vi "NMLWSD_Stability_Data_Collection.vi"() -> ()   [LabVIEW 2017]
uses:
  C:/Program Files (x86)/Newport/Newport USB Driver/Bin/UsbDllWrap.dll
  Program Files (x86)/Newport/Newport USB Driver/Bin/UsbDllWrap.dll
  <vilib>/Analysis/baseanly.llb/Mean (DBL).vi
  <vilib>/Utility/file.llb/Write Delimited Spreadsheet (string).vi
  <vilib>/Analysis/NI_AALBase.lvlib
panel:
  in  "Time":refnum<vi>
  in  "Date":refnum<vi>
  in  "Bytes Received":refnum<vi>
  in  "Module Error":refnum<vi>
  in  "Read Buffer":refnum<vi>
  out "read buffer":string
  in  "Error Log Msg":refnum<vi>
  out "System Data Array":dbl[][](array[numeric])
  out "MCU Data Array":dbl[][](array[numeric])
  in  "Data Error":refnum<vi>
  in  "TimeOut Error":refnum<vi>
  in  "Status Msg":refnum<vi>
  in  "Shutter Closed":refnum<vi>
  in  "Shutter Opened":refnum<vi>
  in  "Active UUT COMs":refnum<visa-resource-name>[](array[refnum])
  in  "Power Meter Ref":refnum<k24>
  out "Shtr Close":bool
  out "Shtr Open":bool
  out "All Results":dbl[][][](array[numeric]) format="%8_4g"
  in  "Serial Number":string[](array[string])=["1"]
  in  "Tpass Shtr Open":bool
  out "Shtr Ref Time":timestamp
  out "TimeS":string caption="Time"
  out "DateS":string caption="Date"
  out "Msg":string="\n\r" caption="Status"
  out "Bytes Rcvd":u32=1000
  out "Module Error":bool[](array[boolean])
  out "Data Error":bool
  out "Timeout":bool
  out "Points":i32[](array[numeric])
  out "UUT Count":i32(ring)=1 items=["1"=1, "2"=2, "3"=3, "4"=4, "5"=5, "6"=6, "7"=7, "8"=8]
  out "error":errorcluster
  out "Data Time":timestamp
  out "Collect":bool
  out "Save":bool
  out "Update Graph":bool
  in  "cDAQ2":string
  in  "Meas N":i32
  in  "WL: NML Only":i32(ring) items=["Red Only", "IR"]
  in  "FW inTest":u16(ring) items=["WSD Board", "NML Board"]
  in  "Sys Criteria":string[][](array[string])
  in  "FW Criteria":string[][](array[string])
  in  "FW ID":string[](array[string])
  in  "FW Prm":string[](array[string])
  out "SysCheck":string[][](array[string])
  out "MCUCheck":string[][](array[string])
  out "SysTrue":bool[][](array[boolean])
  out "MCUTrue":bool[][](array[boolean])
  in  "Shtr Ctrl Close, Seconds":dbl=6.0 max=60.0 format="%.3f"
  in  "cDAQ1":string
  out "Error Log Msg":string
  out "work buffer":string
  in  "Log File":path=path "C:/Test/WSNM Stability/Log.txt"
  out "System Data":dbl[](array[numeric]) format="%#_5p"
  out "MCU Data":dbl[](array[numeric]) format="%#_5p"
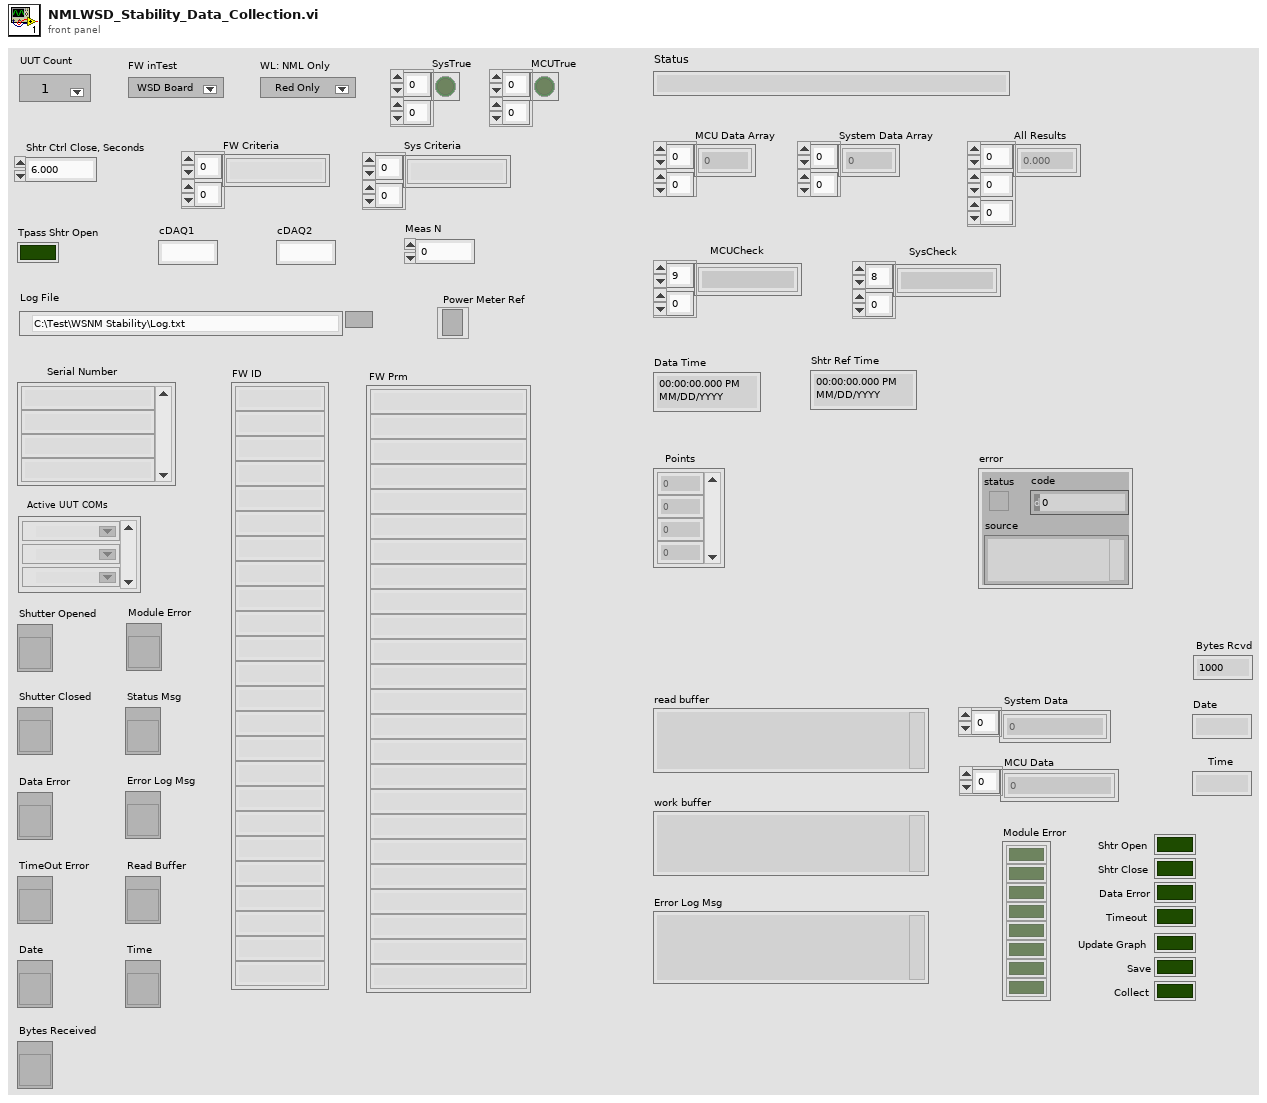
[diagram p1: front panel]
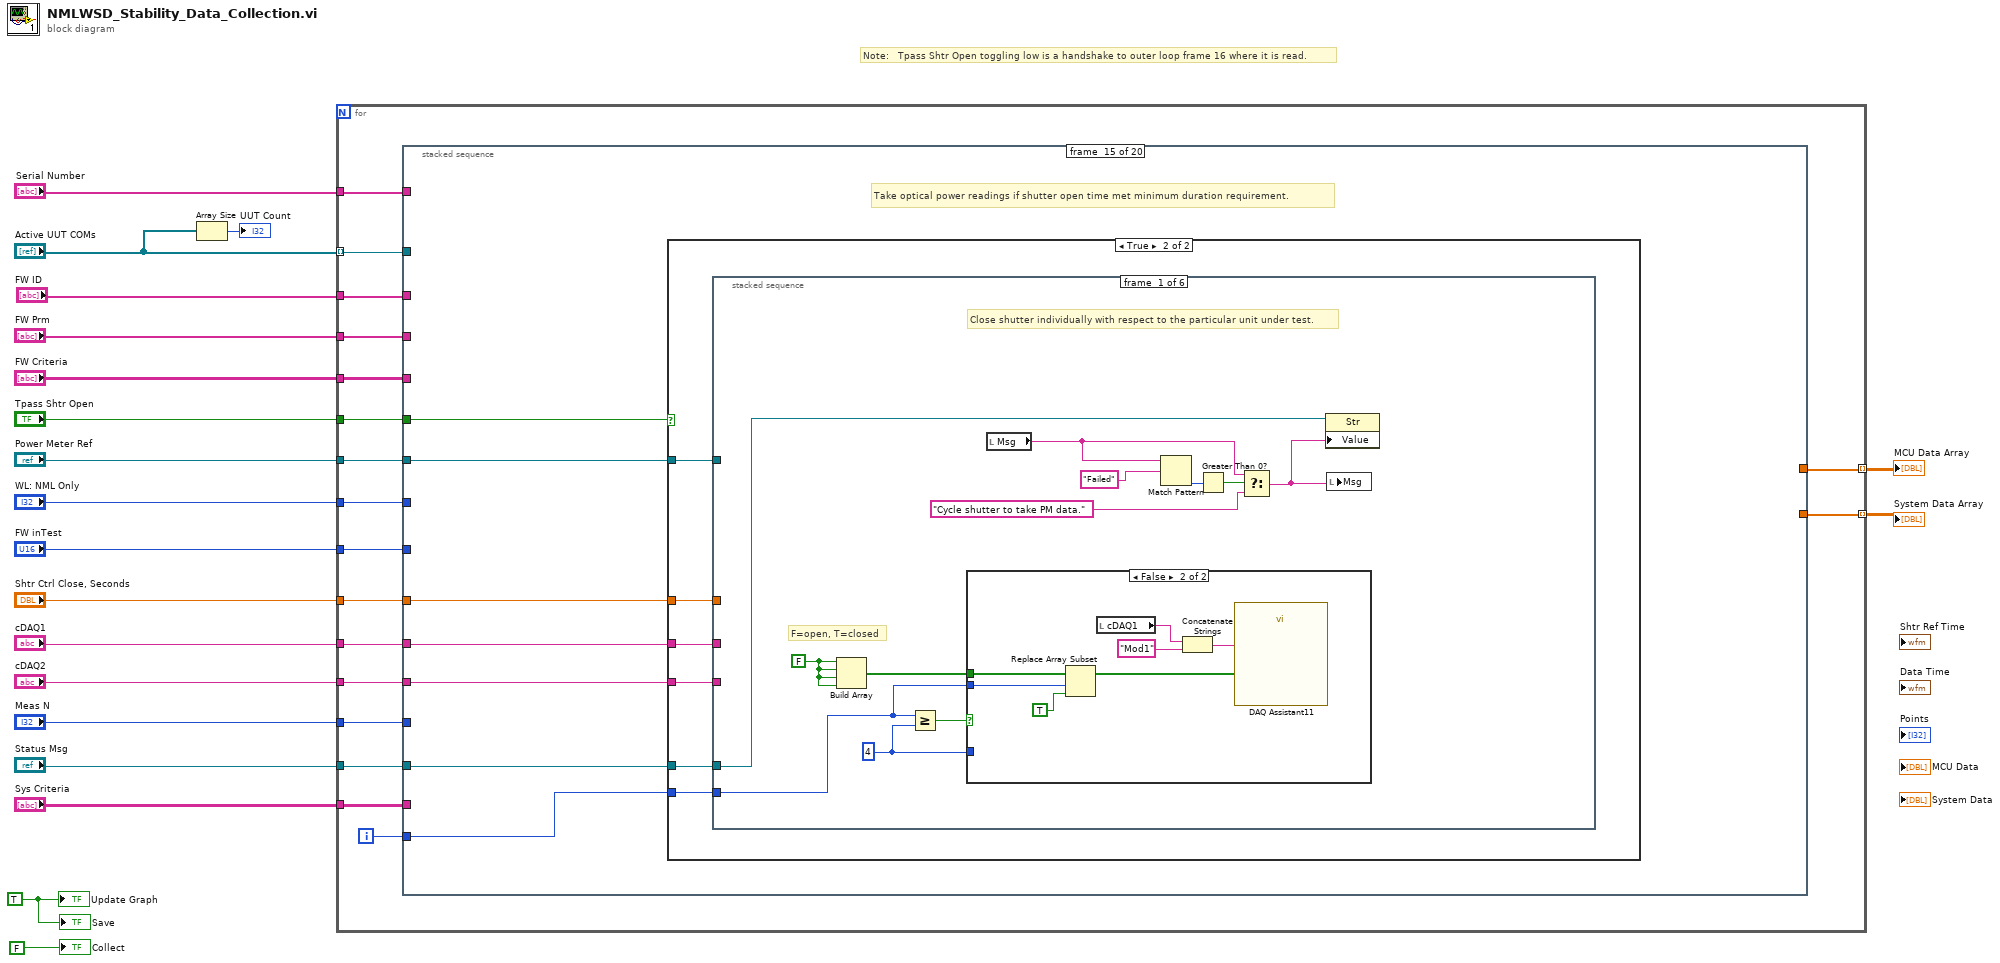
[diagram p0: block diagram]
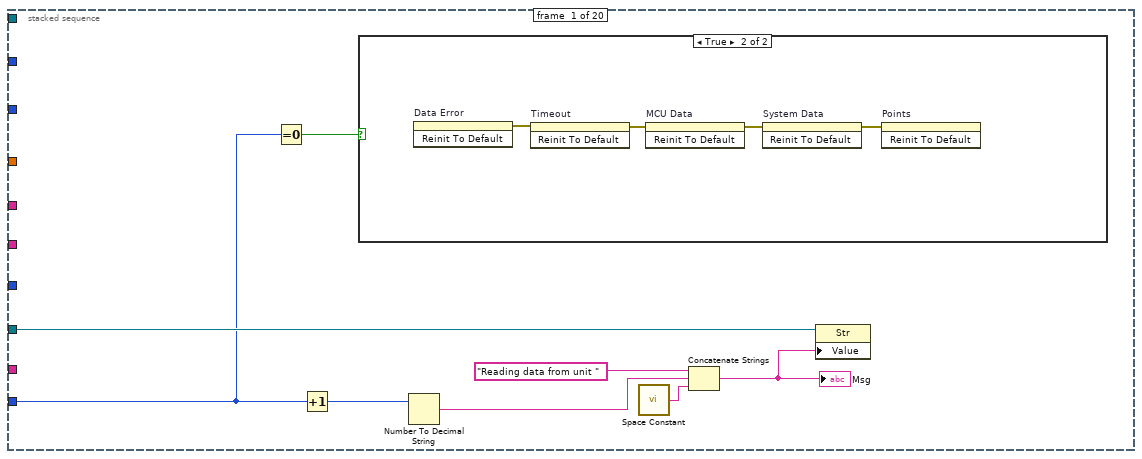
[diagram p2: hidden frame]
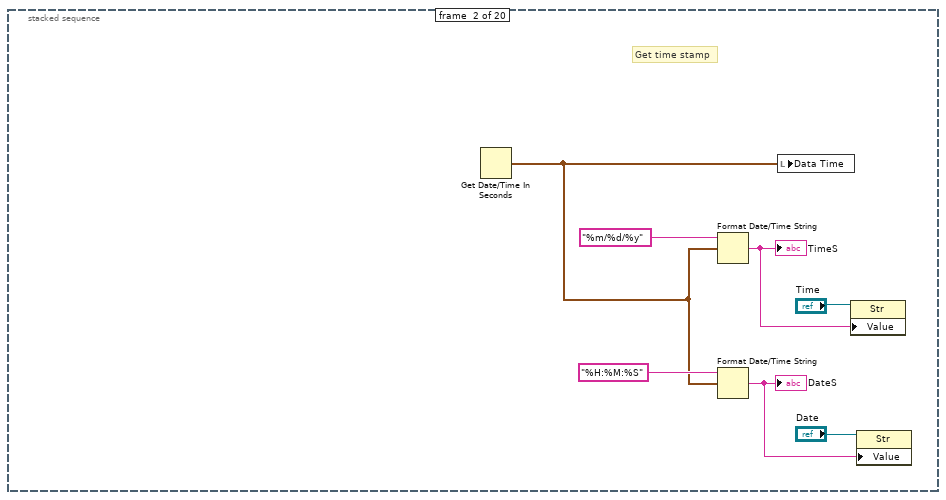
[diagram p4: hidden frame]
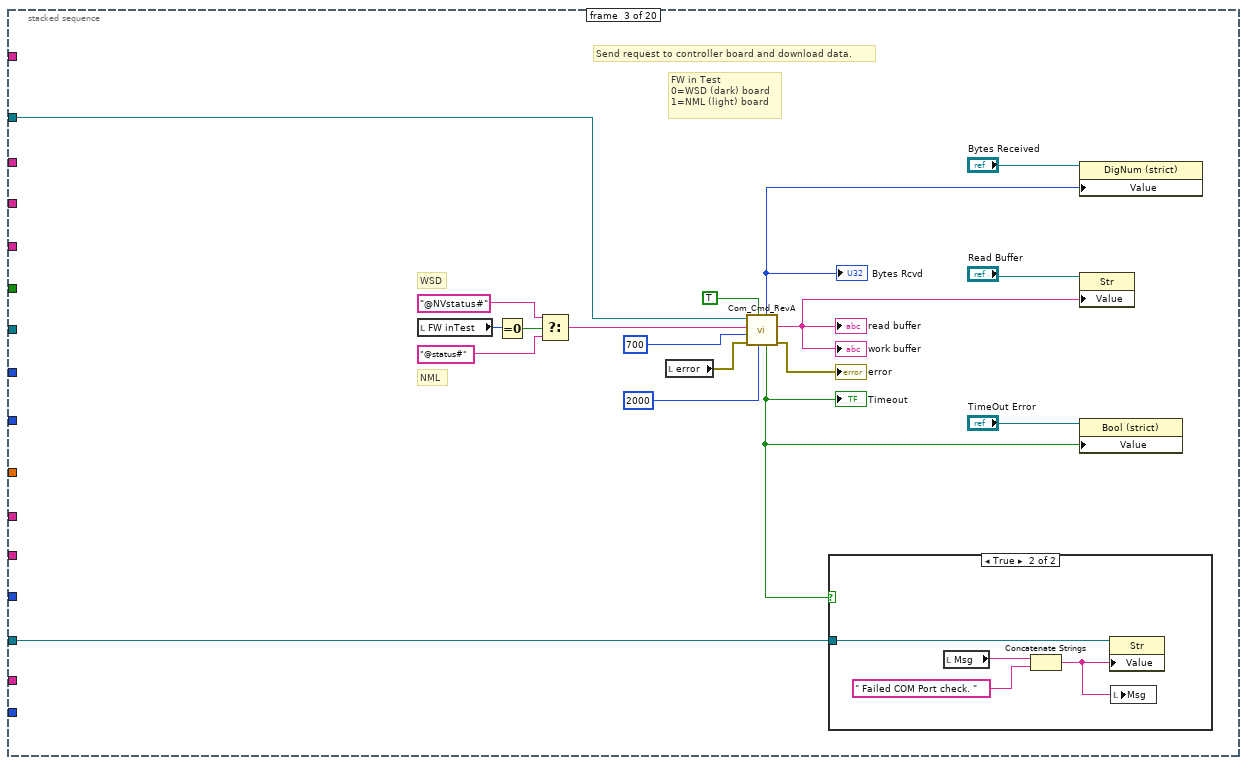
[diagram p5: hidden frame]
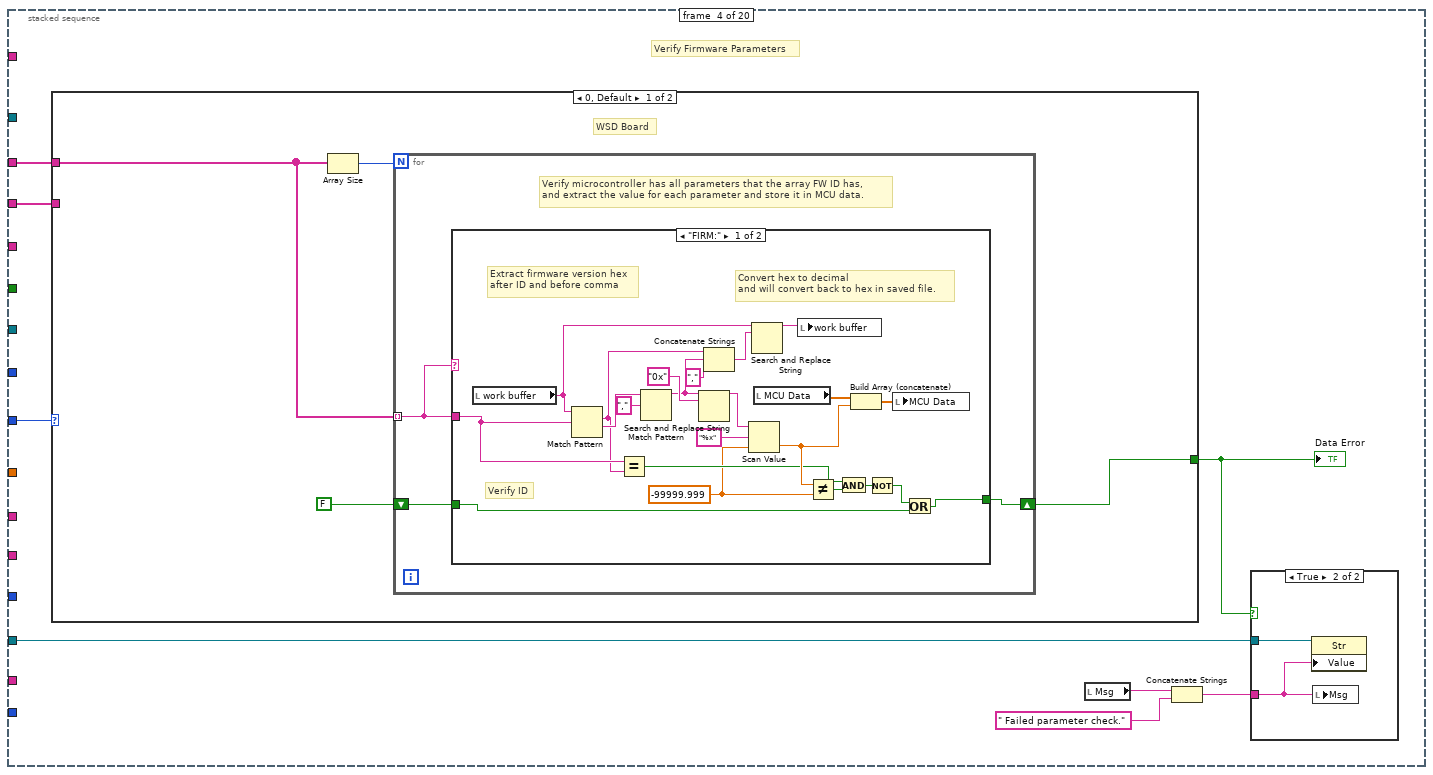
[diagram p7: hidden frame]
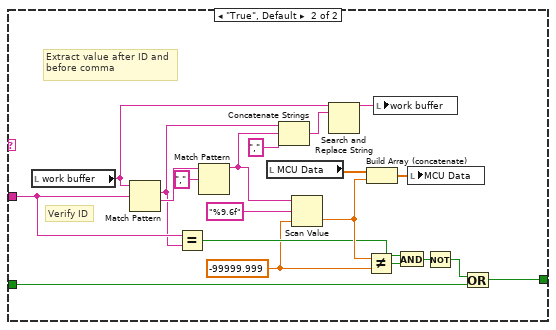
[diagram p9: hidden frame]
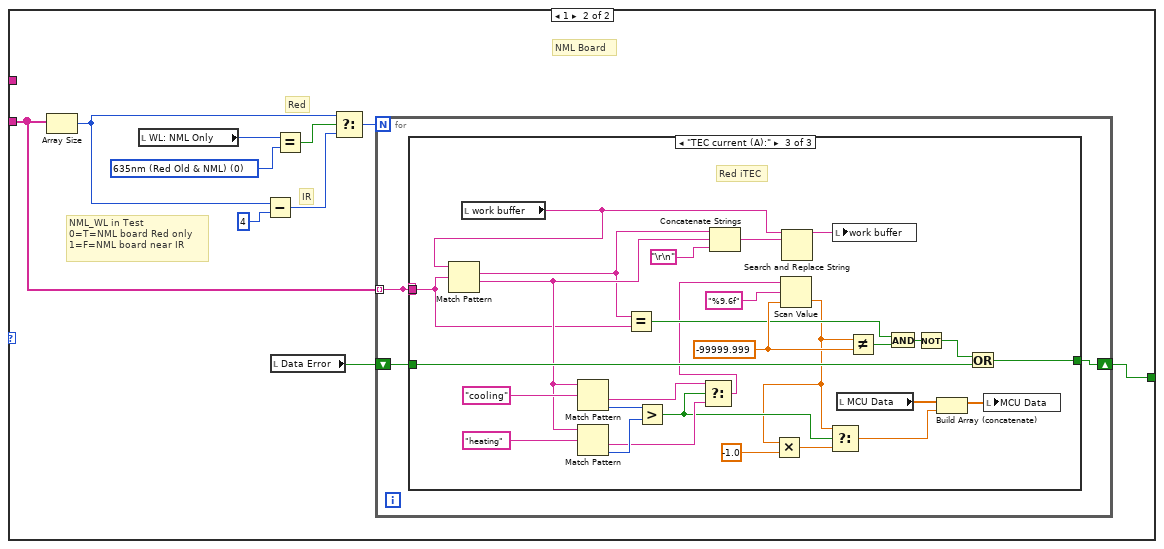
[diagram p10: hidden frame]
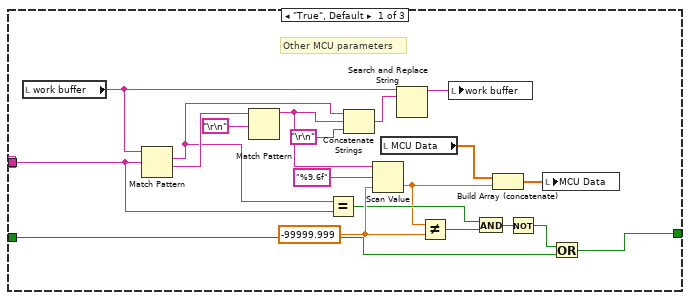
[diagram p11: hidden frame]
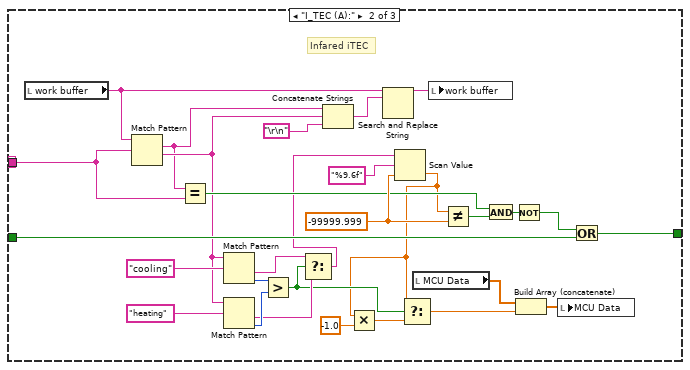
[diagram p12: hidden frame]
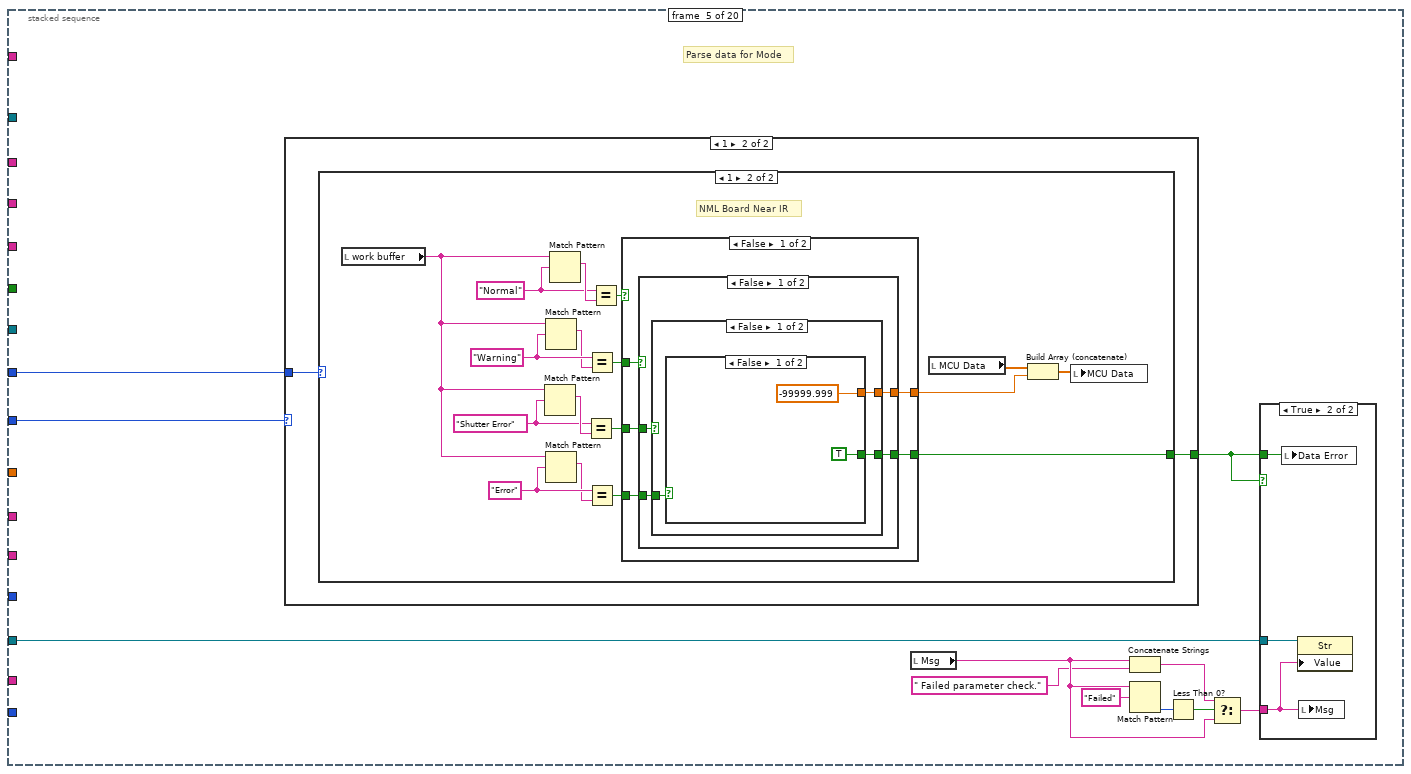
[diagram p13: hidden frame]
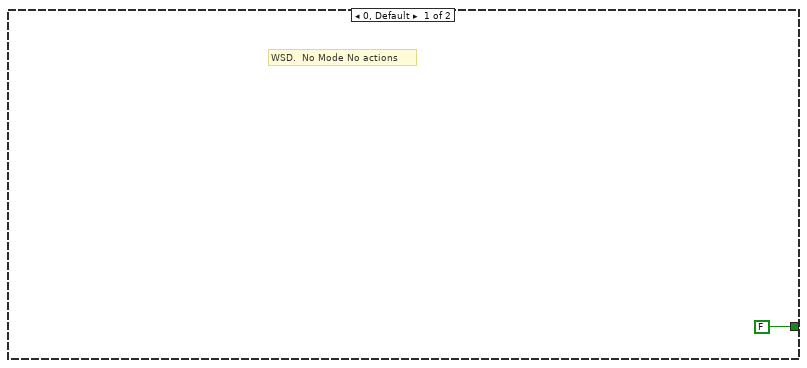
[diagram p15: hidden frame]
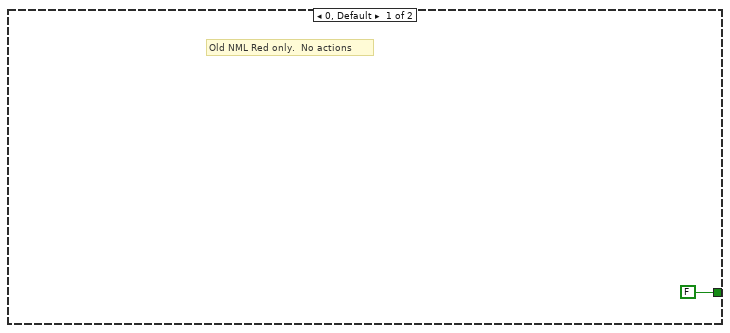
[diagram p16: hidden frame]
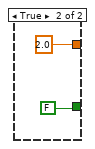
[diagram p17: hidden frame]
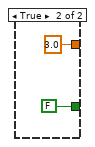
[diagram p18: hidden frame]
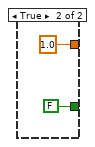
[diagram p19: hidden frame]
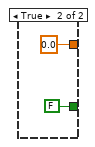
[diagram p20: hidden frame]
diagram:
  w20 = TRUE ("Update Graph")
  # "Note:   Tpass Shtr Open toggling low is a handshake to outer loop frame 16 where it is read."
  n1 = Array Size(array="Active UUT COMs") -> (size(s)=→"UUT Count":i32)
  n2 = for {
    tunnel: "Active UUT COMs" -> [w37] mode=indexing
    tunnel: "Power Meter Ref" -> [w36]
    tunnel: "Tpass Shtr Open" -> [w35]
    tunnel: "FW inTest" -> [w34]
    tunnel: "WL: NML Only" -> [w33]
    tunnel: "Shtr Ctrl Close, Seconds" -> [w32]
    tunnel: "cDAQ1" -> [w31]
    tunnel: "cDAQ2" -> [w30]
    tunnel: "FW ID" -> [w29]
    tunnel: "Meas N" -> [w28]
    tunnel: "Serial Number" -> [w27]
    tunnel: "Status Msg" -> [w26]
    tunnel: "Sys Criteria" -> [w25]
    tunnel: "FW Criteria" -> [w24]
    tunnel: [w23] -> w3 mode=indexing
    tunnel: [w22] -> w2 mode=indexing
    tunnel: "FW Prm" -> [w21]
    i -> [w38]
    n3 = stacked-sequence {
      tunnel: w38 -> [w43 _ _ _ _ _ _ w394 _ w442 _ _ _ w496 w573 w673 w693 w703 w744 _]
      tunnel: w37 -> [_ _ w65 _ _ _ _ _ _ _ _ _ _ _ _ _ _ _ _ _]
      tunnel: w36 -> [_ _ _ _ _ _ _ _ _ w441 _ _ _ _ w572 _ _ _ _ _]
      tunnel: w35 -> [_ _ _ _ _ _ _ _ _ _ _ _ _ _ w571 _ _ _ _ _]
      tunnel: w34 -> [_ _ _ w87 w240 w297 w354 _ _ _ _ _ _ _ _ _ _ _ _ _]
      tunnel: w33 -> [_ _ _ _ w239 w296 w353 _ _ _ _ _ _ _ _ _ _ _ _ _]
      tunnel: w32 -> [_ _ _ _ _ _ _ _ _ _ _ _ _ _ w570 _ _ _ _ _]
      tunnel: w31 -> [_ _ _ _ _ _ _ _ _ _ _ w471 _ _ w569 _ _ _ _ _]
      tunnel: w30 -> [_ _ _ _ _ _ _ _ _ _ _ _ _ _ w568 _ _ _ _ _]
      tunnel: w29 -> [_ _ _ w86 _ _ _ _ _ _ _ _ _ _ _ _ _ _ _ _]
      tunnel: w28 -> [_ _ _ _ _ _ _ _ _ _ _ _ _ _ _ w672 _ _ _ _]
      tunnel: w27 -> [_ _ _ _ _ _ _ w392 _ _ _ _ _ _ _ _ _ _ _ _]
      tunnel: w26 -> [w45 _ w63 w82 w232 w289 w346 _ w434 _ w465 _ w489 _ w567 _ _ _ _ _]
      tunnel: w25 -> [_ _ _ _ _ _ _ _ _ _ _ _ _ _ _ _ _ w702 _ _]
      tunnel: w24 -> [_ _ _ _ _ _ _ _ _ _ _ _ _ _ _ _ _ w701 _ _]
      tunnel: [_ _ _ _ _ _ _ _ _ _ _ _ _ _ _ _ w691 _ _ _] -> w23
      tunnel: [_ _ _ _ _ _ _ _ _ _ _ _ _ _ _ _ w690 _ _ _] -> w22
      tunnel: w21 -> [_ _ _ w80 _ _ _ _ _ _ _ _ _ _ _ _ _ _ _ _]
      frame #0 {
        n4 = Equal To 0?(x=w43) -> (x = 0?=w46:bool)
        n5 = Increment(x=w43) -> (x+1=w44:i32)
        n6 = case shown="True" w46 {
          frame False {
          }
          frame True {
            n7 = invoke on="Data Error" class="Bool (strict)" method="Reinit To Default"() -> (error out=w49:errorcluster)  [unwired: 3 in, 2 out]
            n8 = invoke on="Timeout" class="Bool (strict)" method="Reinit To Default"(error in=w49) -> (error out=w48:errorcluster)  [unwired: 2 in, 2 out]
            n9 = invoke on="MCU Data" class="Arr (strict)" method="Reinit To Default"(error in=w48) -> (error out=w50:errorcluster)  [unwired: 2 in, 2 out]
            n10 = invoke on="System Data" class="Arr (strict)" method="Reinit To Default"(error in=w50) -> (error out=w47:errorcluster)  [unwired: 2 in, 2 out]
            n11 = invoke on="Points" class="Arr (strict)" method="Reinit To Default"(error in=w47) -> ()  [unwired: 2 in, 3 out]
          }
        }
        n12 = Number To Decimal String(number=w44) -> (decimal integer string=w41:string)  [unwired: 1 in]
        n13 = call <vilib>:"Space Constant.vi"() -> ("String"=w39:string)
        n14 = Concatenate Strings("Reading data from unit " ("Msg"), w41, w39) -> (w40:string)
        "Msg" <- w40
        n15 = property class="Str"(reference=w45, "Value"=w40) -> ()  [unwired: 1 in, 2 out]
      }
      frame #1 {
        # "Get time stamp"
        n16 = Get Date/Time In Seconds() -> (seconds since 1Jan1904=w55:timestamp)
        n17 = Format Date/Time String(time format string (%c)="%m/%d/%y", seconds (now)=w55) -> (date/time string=w52:string)  [unwired: 1 in]
        "TimeS" <- w52
        n18 = Format Date/Time String(time format string (%c)="%H:%M:%S", seconds (now)=w55) -> (date/time string=w51:string)  [unwired: 1 in]
        "DateS" <- w51
        n19 = local write "Data Time"(w55) -> ()
        n20 = property class="Str"(reference="Time", "Value"=w52) -> ()  [unwired: 1 in, 2 out]
        n21 = property class="Str"(reference="Date", "Value"=w51) -> ()  [unwired: 1 in, 2 out]
      }
      frame #2 {
        # "NML"
        # "WSD"
        # "FW in Test\n0=WSD (dark) board\n1=NML (light) board"
        # "Send request to controller board and download data."
        n22 = local read "FW inTest"() -> (w68:u16)
        n23 = Equal To 0?(x=w68) -> (x = 0?=w67:bool)
        n24 = Select(t="@NVstatus#" ("string"), s=w67, f="@status#" ("string")) -> (s? t:f=w71:string)
        n25 = local read "error"() -> (w75:errorcluster)
        n26 = call "Com_Cmd_RevA.vi"("Timeout"=2000, "Query"=TRUE, "error in"=w75, "Delay, ms"=u32 700, "write buffer"=w71, "VISA"=w65) -> ("error out"=→"error":errorcluster, "read buffer"=w60:string, "Timeout"=w62:bool, "return count"=w58:u32)  [unwired: 2 out]
        "work buffer" <- w60
        "Timeout" <- w62
        "Bytes Rcvd" <- w58
        "read buffer" <- w60
        n27 = case shown="True" w62 {
          tunnel: w63 -> [_ w77]
          frame False {
          }
          frame True {
            n28 = local read "Msg"() -> (w79:string)
            n29 = Concatenate Strings(w79, " Failed COM Port check. " ("string")) -> (w76:string)
            n30 = property class="Str"(reference=w77, "Value"=w76) -> ()  [unwired: 1 in, 2 out]
            n31 = local write "Msg"(w76) -> ()
          }
        }
        n32 = property class="DigNum (strict)"(reference="Bytes Received", "Value"=w58) -> ()  [unwired: 1 in, 2 out]
        n33 = property class="Str"(reference="Read Buffer", "Value"=w60) -> ()  [unwired: 1 in, 2 out]
        n34 = property class="Bool (strict)"(reference="TimeOut Error", "Value"=w62) -> ()  [unwired: 1 in, 2 out]
      }
      frame #3 {
        # "Verify Firmware Parameters"
        n35 = case shown="0, Default" w87 {
          tunnel: w86 -> [w91 _]
          tunnel: [w90 w140] -> w85
          tunnel: w80 -> [_ w139]
          frame 0, Default {
            # "WSD Board"
            n36 = Array Size(array=w91) -> (size(s)=w92:i32)
            n37 = for {
              N: w92 -> [_]
              shift-right: [w95] -> w90
              shift-left: FALSE ("Data Err") -> [w96]
              tunnel: w91 -> [w94] mode=indexing
              # "Verify microcontroller has all parameters that the array FW ID has,\nand extract the value for each parameter and store it in MCU data."
              n38 = case shown="\"FIRM:\"" w94 {
                tunnel: w94 -> [w105 w125]
                tunnel: w96 -> [w107 w138]
                tunnel: [w106 w137] -> w95
                frame "FIRM:" {
                  w111 = -99999.999 ("default (0 dbl)")
                  # "Convert hex to decimal\nand will convert back to hex in saved file."
                  # "Extract firmware version hex\nafter ID and before comma"
                  # "Verify ID"
                  n39 = local read "work buffer"() -> (w99:string)
                  n40 = Match Pattern(string=w99, regular expression=w105) -> (match substring=w102:string, after substring=w109:string)  [unwired: 1 in, 2 out]
                  n41 = Equal?(x=w105, y=w102) -> (x = y?=w113:bool)
                  n42 = Match Pattern(string=w109, regular expression=",") -> (before substring=w101:string)  [unwired: 1 in, 3 out]
                  n43 = Search and Replace String(input string=w101, search string="0x") -> (result string=w103:string)  [unwired: 6 in, 3 out]
                  n44 = Concatenate Strings(w102, w101, "," ("string")) -> (w98:string)
                  n45 = Scan Value(string=w103, format string="%x", default (0 dbl)=w111) -> (value=w116:dbl)  [unwired: 1 out]
                  n46 = Search and Replace String(input string=w99, search string=w98) -> (result string=w97:string)  [unwired: 6 in, 3 out]
                  n47 = local read "MCU Data"() -> (w114:dbl[])
                  n48 = local write "work buffer"(w97) -> ()
                  n49 = Not Equal?(x=w116, y=w111) -> (x != y?=w112:bool)
                  n50 = And(x=w113, y=w112) -> (x .and. y?=w117:bool)
                  n51 = Build Array (concatenate)(w114, w116) -> (w115:dbl[])
                  n52 = Not(x=w117) -> (.not. x?=w118:bool)
                  n53 = local write "MCU Data"(w115) -> ()
                  n54 = Or(x=w118, y=w107) -> (x .or. y?=w106:bool)
                }
                frame "True", Default {
                  w129 = -99999.999 ("default (0 dbl)")
                  # "Extract value after ID and\nbefore comma"
                  # "Verify ID"
                  n55 = local read "work buffer"() -> (w121:string)
                  n56 = Match Pattern(string=w121, regular expression=w125) -> (match substring=w123:string, after substring=w127:string)  [unwired: 1 in, 2 out]
                  n57 = Equal?(x=w125, y=w123) -> (x = y?=w131:bool)
                  n58 = Match Pattern(string=w127, regular expression=",") -> (before substring=w122:string)  [unwired: 1 in, 3 out]
                  n59 = local read "MCU Data"() -> (w132:dbl[])
                  n60 = Concatenate Strings(w123, w122, "," ("string")) -> (w120:string)
                  n61 = Scan Value(string=w122, format string="%9.6f", default (0 dbl)=w129) -> (value=w134:dbl)  [unwired: 1 out]
                  n62 = Search and Replace String(input string=w121, search string=w120) -> (result string=w119:string)  [unwired: 6 in, 3 out]
                  n63 = Not Equal?(x=w134, y=w129) -> (x != y?=w130:bool)
                  n64 = Build Array (concatenate)(w132, w134) -> (w133:dbl[])
                  n65 = local write "work buffer"(w119) -> ()
                  n66 = And(x=w131, y=w130) -> (x .and. y?=w135:bool)
                  n67 = local write "MCU Data"(w133) -> ()
                  n68 = Not(x=w135) -> (.not. x?=w136:bool)
                  n69 = Or(x=w136, y=w138) -> (x .or. y?=w137:bool)
                }
              }
            }
          }
          frame 1 {
            w142 = 0 items=["635nm (Red Old & NML)", "Red-780-850nm (IR NewNML FW)", "Mix NML FW"] ("Color")
            # "NML Board"
            # "NML_WL in Test\n0=T=NML board Red only\n1=F=NML board near IR"
            # "IR"
            # "Red"
            n70 = Array Size(array=w139) -> (size(s)=w146:i32)
            n71 = local read "WL: NML Only"() -> (w143:i32)
            n72 = Subtract(x=w146, y=4) -> (x-y=w144:i32)
            n73 = local read "Data Error"() -> (w141:bool)
            n74 = Equal?(x=w143, y=w142) -> (x = y?=w148:bool)
            n75 = Select(t=w146, s=w148, f=w144) -> (s? t:f=w147:i32)
            n76 = for {
              N: w147 -> [_]
              tunnel: w139 -> [w149] mode=indexing
              shift-right: [w150] -> w140
              shift-left: w141 -> [w151]
              n77 = case shown="\"TEC current (A):\"" w149 {
                tunnel: w151 -> [w162 w192 w221]
                tunnel: [w161 w191 w220] -> w150
                tunnel: w149 -> [w153 w172 w202]
                frame "True", Default {
                  w170 = -99999.999 ("default (0 dbl)")
                  # "Other MCU parameters"
                  n78 = local read "work buffer"() -> (w152:string)
                  n79 = Match Pattern(string=w152, regular expression=w153) -> (match substring=w154:string, after substring=w159:string)  [unwired: 1 in, 2 out]
                  n80 = Match Pattern(string=w159, regular expression="\r\n") -> (before substring=w157:string)  [unwired: 1 in, 3 out]
                  n81 = Equal?(x=w154, y=w153) -> (x = y?=w168:bool)
                  n82 = Concatenate Strings(w154, w157, "\r\n") -> (w156:string)
                  n83 = Scan Value(string=w157, format string="%9.6f", default (0 dbl)=w170) -> (value=w165:dbl)  [unwired: 1 out]
                  n84 = local read "MCU Data"() -> (w167:dbl[])
                  n85 = Search and Replace String(input string=w152, search string=w156) -> (result string=w155:string)  [unwired: 6 in, 3 out]
                  n86 = Not Equal?(x=w165, y=w170) -> (x != y?=w169:bool)
                  n87 = local write "work buffer"(w155) -> ()
                  n88 = And(x=w168, y=w169) -> (x .and. y?=w164:bool)
                  n89 = Build Array (concatenate)(w167, w165) -> (w166:dbl[])
                  n90 = Not(x=w164) -> (.not. x?=w163:bool)
                  n91 = local write "MCU Data"(w166) -> ()
                  n92 = Or(x=w163, y=w162) -> (x .or. y?=w161:bool)
                }
                frame "I_TEC (A):" {
                  w199 = -99999.999 ("default (0 dbl)")
                  # "Infared iTEC"
                  n93 = local read "work buffer"() -> (w176:string)
                  n94 = Match Pattern(string=w176, regular expression=w172) -> (match substring=w173:string, after substring=w174:string)  [unwired: 1 in, 2 out]
                  n95 = Equal?(x=w173, y=w172) -> (x = y?=w197:bool)
                  n96 = Match Pattern(string=w174, regular expression="cooling") -> (after substring=w186:string, offset past match=w188:i32)  [unwired: 1 in, 2 out]
                  n97 = Match Pattern(string=w174, regular expression="heating") -> (after substring=w185:string, offset past match=w187:i32)  [unwired: 1 in, 2 out]
                  n98 = Greater?(x=w188, y=w187) -> (0:w184:bool)
                  n99 = Select(t=w186, s=w184, f=w185) -> (s? t:f=w175:string)
                  n100 = Concatenate Strings(w173, w174, "\r\n") -> (w179:string)
                  n101 = Search and Replace String(input string=w176, search string=w179) -> (result string=w178:string)  [unwired: 6 in, 3 out]
                  n102 = Scan Value(string=w175, format string="%9.6f", default (0 dbl)=w199) -> (value=w181:dbl)  [unwired: 1 out]
                  n103 = Multiply(x=w181, y=-1.0) -> (x*y=w182:dbl)
                  n104 = Select(t=w181, s=w184, f=w182) -> (s? t:f=w180:dbl)
                  n105 = local read "MCU Data"() -> (w196:dbl[])
                  n106 = local write "work buffer"(w178) -> ()
                  n107 = Not Equal?(x=w181, y=w199) -> (x != y?=w198:bool)
                  n108 = And(x=w197, y=w198) -> (x .and. y?=w194:bool)
                  n109 = Not(x=w194) -> (.not. x?=w193:bool)
                  n110 = Build Array (concatenate)(w196, w180) -> (w195:dbl[])
                  n111 = local write "MCU Data"(w195) -> ()
                  n112 = Or(x=w193, y=w192) -> (x .or. y?=w191:bool)
                }
                frame "TEC current (A):" {
                  w228 = -99999.999 ("default (0 dbl)")
                  # "Red iTEC"
                  n113 = local read "work buffer"() -> (w204:string)
                  n114 = Match Pattern(string=w204, regular expression=w202) -> (match substring=w201:string, after substring=w203:string)  [unwired: 1 in, 2 out]
                  n115 = Match Pattern(string=w203, regular expression="cooling") -> (after substring=w215:string, offset past match=w217:i32)  [unwired: 1 in, 2 out]
                  n116 = Match Pattern(string=w203, regular expression="heating") -> (after substring=w214:string, offset past match=w216:i32)  [unwired: 1 in, 2 out]
                  n117 = Equal?(x=w201, y=w202) -> (x = y?=w226:bool)
                  n118 = Greater?(x=w217, y=w216) -> (0:w212:bool)
                  n119 = Select(t=w215, s=w212, f=w214) -> (s? t:f=w213:string)
                  n120 = Concatenate Strings(w201, w203, "\r\n") -> (w207:string)
                  n121 = Scan Value(string=w213, format string="%9.6f", default (0 dbl)=w228) -> (value=w209:dbl)  [unwired: 1 out]
                  n122 = Multiply(x=w209, y=-1.0) -> (x*y=w210:dbl)
                  n123 = Search and Replace String(input string=w204, search string=w207) -> (result string=w206:string)  [unwired: 6 in, 3 out]
                  n124 = Select(t=w209, s=w212, f=w210) -> (s? t:f=w208:dbl)
                  n125 = local write "work buffer"(w206) -> ()
                  n126 = local read "MCU Data"() -> (w225:dbl[])
                  n127 = Not Equal?(x=w209, y=w228) -> (x != y?=w227:bool)
                  n128 = And(x=w226, y=w227) -> (x .and. y?=w223:bool)
                  n129 = Not(x=w223) -> (.not. x?=w222:bool)
                  n130 = Build Array (concatenate)(w225, w208) -> (w224:dbl[])
                  n131 = Or(x=w222, y=w221) -> (x .or. y?=w220:bool)
                  n132 = local write "MCU Data"(w224) -> ()
                }
              }
            }
          }
        }
        "Data Error" <- w85
        n133 = local read "Msg"() -> (w84:string)
        n134 = Concatenate Strings(w84, " Failed parameter check." ("string")) -> (w81:string)
        n135 = case shown="True" w85 {
          tunnel: w82 -> [_ w89]
          tunnel: w81 -> [_ w88]
          frame False {
          }
          frame True {
            n136 = property class="Str"(reference=w89, "Value"=w88) -> ()  [unwired: 1 in, 2 out]
            n137 = local write "Msg"(w88) -> ()
          }
        }
      }
      frame #4 {
        # "Parse data for Mode"
        n138 = case shown="1" w240 {
          tunnel: w239 -> [_ w246]
          tunnel: [FALSE w245] -> w231
          frame 0, Default {
            # "WSD.  No Mode No actions"
          }
          frame 1 {
            n139 = case shown="1" w246 {
              tunnel: [FALSE w248] -> w245
              frame 0, Default {
                # "Old NML Red only.  No actions"
              }
              frame 1 {
                w256 = "Error" ("regular expression")
                w257 = "Shutter Error" ("regular expression")
                w260 = "Warning" ("regular expression")
                w261 = "Normal" ("regular expression")
                # "NML Board Near IR"
                n140 = local read "work buffer"() -> (w254:string)
                n141 = Match Pattern(string=w254, regular expression=w257) -> (match substring=w258:string)  [unwired: 1 in, 3 out]
                n142 = Match Pattern(string=w254, regular expression=w260) -> (match substring=w259:string)  [unwired: 1 in, 3 out]
                n143 = Match Pattern(string=w254, regular expression=w256) -> (match substring=w255:string)  [unwired: 1 in, 3 out]
                n144 = Match Pattern(string=w254, regular expression=w261) -> (match substring=w264:string)  [unwired: 1 in, 3 out]
                n145 = Equal?(x=w257, y=w258) -> (x = y?=w250:bool)
                n146 = Equal?(x=w260, y=w259) -> (x = y?=w251:bool)
                n147 = Equal?(x=w256, y=w255) -> (x = y?=w249:bool)
                n148 = Equal?(x=w261, y=w264) -> (x = y?=w253:bool)
                n149 = case shown="False" w253 {
                  tunnel: [w268 0.0] -> w252
                  tunnel: w251 -> [w269 _]
                  tunnel: w250 -> [w267 _]
                  tunnel: w249 -> [w266 _]
                  tunnel: [w265 FALSE] -> w248
                  frame False {
                    n150 = case shown="False" w269 {
                      tunnel: [w272 1.0] -> w268
                      tunnel: w267 -> [w273 _]
                      tunnel: w266 -> [w271 _]
                      tunnel: [w270 FALSE] -> w265
                      frame False {
                        n151 = case shown="False" w273 {
                          tunnel: [w275 3.0] -> w272
                          tunnel: w271 -> [w276 _]
                          tunnel: [w274 FALSE] -> w270
                          frame False {
                            n152 = case shown="False" w276 {
                              tunnel: [-99999.999 ("default (0 dbl)") 2.0] -> w275
                              tunnel: [TRUE ("Data Err") FALSE] -> w274
                              frame False {
                              }
                              frame True {
                              }
                            }
                          }
                          frame True {
                          }
                        }
                      }
                      frame True {
                      }
                    }
                  }
                  frame True {
                  }
                }
                n153 = local read "MCU Data"() -> (w263:dbl[])
                n154 = Build Array (concatenate)(w263, w252) -> (w262:dbl[])
                n155 = local write "MCU Data"(w262) -> ()
              }
            }
          }
        }
        n156 = local read "Msg"() -> (w237:string)
        n157 = Concatenate Strings(w237, " Failed parameter check." ("string")) -> (w236:string)
        n158 = Match Pattern(string=w237, regular expression="Failed") -> (offset past match=w234:i32)  [unwired: 1 in, 3 out]
        n159 = Less Than 0?(x=w234) -> (x < 0?=w235:bool)
        n160 = Select(t=w236, s=w235, f=w237) -> (s? t:f=w238:string)
        n161 = case shown="True" w231 {
          tunnel: w232 -> [_ w243]
          tunnel: w238 -> [_ w242]
          tunnel: w231 -> [_ w241]
          frame False {
          }
          frame True {
            n162 = local write "Data Error"(w241) -> ()
            n163 = property class="Str"(reference=w243, "Value"=w242) -> ()  [unwired: 1 in, 2 out]
            n164 = local write "Msg"(w242) -> ()
          }
        }
      }
      frame #5 {
        # "Parse data for wavelength."
        n165 = case shown="1" w297 {
          tunnel: w296 -> [_ w303]
          tunnel: [FALSE w302] -> w288
          frame 0, Default {
            # "WSD.  No Mode No actions"
          }
          frame 1 {
            # "NML_WL in Test\n0=T=NML board Red only\n1=F=NML board near IR"
            # "NML"
            n166 = case shown="1" w303 {
              tunnel: [FALSE w305] -> w302
              frame 0, Default {
                # "Old NML Red only.  No actions"
              }
              frame 1 {
                w313 = "850" ("regular expression")
                w314 = "780" ("regular expression")
                w317 = "Red" ("regular expression")
                w318 = "None" ("regular expression")
                # "NML IR"
                n167 = local read "work buffer"() -> (w311:string)
                n168 = Match Pattern(string=w311, regular expression=w314) -> (match substring=w315:string)  [unwired: 1 in, 3 out]
                n169 = Match Pattern(string=w311, regular expression=w317) -> (match substring=w316:string)  [unwired: 1 in, 3 out]
                n170 = Match Pattern(string=w311, regular expression=w313) -> (match substring=w312:string)  [unwired: 1 in, 3 out]
                n171 = Match Pattern(string=w311, regular expression=w318) -> (match substring=w321:string)  [unwired: 1 in, 3 out]
                n172 = Equal?(x=w314, y=w315) -> (x = y?=w307:bool)
                n173 = Equal?(x=w317, y=w316) -> (x = y?=w308:bool)
                n174 = Equal?(x=w313, y=w312) -> (x = y?=w306:bool)
                n175 = Equal?(x=w318, y=w321) -> (x = y?=w310:bool)
                n176 = case shown="False" w310 {
                  tunnel: [w325 0.0] -> w309
                  tunnel: w308 -> [w326 _]
                  tunnel: w307 -> [w324 _]
                  tunnel: w306 -> [w323 _]
                  tunnel: [w322 FALSE] -> w305
                  frame False {
                    n177 = case shown="False" w326 {
                      tunnel: [w329 1.0] -> w325
                      tunnel: w324 -> [w330 _]
                      tunnel: w323 -> [w328 _]
                      tunnel: [w327 FALSE] -> w322
                      frame False {
                        n178 = case shown="False" w330 {
                          tunnel: [w332 2.0] -> w329
                          tunnel: w328 -> [w333 _]
                          tunnel: [w331 FALSE] -> w327
                          frame False {
                            n179 = case shown="False" w333 {
                              tunnel: [-99999.999 ("default (0 dbl)") 3.0] -> w332
                              tunnel: [TRUE ("Data Err") FALSE] -> w331
                              frame False {
                              }
                              frame True {
                              }
                            }
                          }
                          frame True {
                          }
                        }
                      }
                      frame True {
                      }
                    }
                  }
                  frame True {
                  }
                }
                n180 = local read "MCU Data"() -> (w320:dbl[])
                n181 = Build Array (concatenate)(w320, w309) -> (w319:dbl[])
                n182 = local write "MCU Data"(w319) -> ()
              }
            }
          }
        }
        n183 = local read "Msg"() -> (w291:string)
        n184 = Concatenate Strings(w291, " Failed parameter check." ("string")) -> (w292:string)
        n185 = Match Pattern(string=w291, regular expression="Failed") -> (offset past match=w295:i32)  [unwired: 1 in, 3 out]
        n186 = Less Than 0?(x=w295) -> (x < 0?=w293:bool)
        n187 = Select(t=w292, s=w293, f=w291) -> (s? t:f=w290:string)
        n188 = case shown="True" w288 {
          tunnel: w289 -> [_ w300]
          tunnel: w290 -> [_ w299]
          tunnel: w288 -> [_ w298]
          frame False {
          }
          frame True {
            n189 = local write "Data Error"(w298) -> ()
            n190 = property class="Str"(reference=w300, "Value"=w299) -> ()  [unwired: 1 in, 2 out]
            n191 = local write "Msg"(w299) -> ()
          }
        }
      }
      frame #6 {
        # "Parse Data for LHM Calibration Gain and Offset"
        n192 = case shown="1" w354 {
          tunnel: w353 -> [_ w360]
          tunnel: [FALSE w359] -> w345
          frame 0, Default {
            # "WSD.  No Mode No actions"
          }
          frame 1 {
            # "NML"
            n193 = case shown="1" w360 {
              tunnel: [FALSE w362] -> w359
              frame 0, Default {
                # "Old NML Red only.  No actions"
              }
              frame 1 {
                w363 = "LHM Calibration:" ("regular expression")
                w370 = -99999.999 ("default (0 dbl)")
                # "NML IR"
                n194 = local read "work buffer"() -> (w377:string)
                n195 = Match Pattern(string=w377, regular expression=w363) -> (match substring=w364:string, after substring=w378:string)  [unwired: 1 in, 2 out]
                n196 = Equal?(x=w364, y=w363) -> (x = y?=w383:bool)
                n197 = Match Pattern(string=w378, regular expression="Gain=") -> (after substring=w373:string)  [unwired: 1 in, 3 out]
                n198 = Match Pattern(string=w378, regular expression="Offset=") -> (after substring=w374:string)  [unwired: 1 in, 3 out]
                n199 = Match Pattern(string=w373, regular expression=",") -> (before substring=w372:string)  [unwired: 1 in, 3 out]
                n200 = Concatenate Strings(w364, w378, "\r\n") -> (w380:string)
                n201 = Search and Replace String(input string=w377, search string=w380) -> (result string=w379:string)  [unwired: 6 in, 3 out]
                n202 = Scan Value(string=w372, format string="%9.6f", default (0 dbl)=w370) -> (value=w385:dbl)  [unwired: 1 out]
                n203 = Scan Value(string=w374, format string="%9.6f", default (0 dbl)=w370) -> (value=w386:dbl)  [unwired: 1 out]
                n204 = local write "work buffer"(w379) -> ()
                n205 = Not Equal?(x=w385, y=w370) -> (x != y?=w384:bool)
                n206 = Not Equal?(x=w386, y=w370) -> (x != y?=w376:bool)
                n207 = Compound Arithmetic op=AND(w383, w384, w376) -> (w375:bool)
                n208 = Not(x=w375) -> (.not. x?=w362:bool)
                n209 = local read "MCU Data"() -> (w382:dbl[])
                n210 = Build Array (concatenate)(w382, w385, w386) -> (w381:dbl[])
                n211 = local write "MCU Data"(w381) -> ()
              }
            }
          }
        }
        n212 = local read "Msg"() -> (w349:string)
        n213 = Concatenate Strings(w349, " Failed parameter check." ("string")) -> (w350:string)
        n214 = Match Pattern(string=w349, regular expression="Failed") -> (offset past match=w352:i32)  [unwired: 1 in, 3 out]
        n215 = Less Than 0?(x=w352) -> (x < 0?=w351:bool)
        n216 = Select(t=w350, s=w351, f=w349) -> (s? t:f=w348:string)
        n217 = case shown="True" w345 {
          tunnel: w346 -> [_ w357]
          tunnel: w348 -> [_ w356]
          tunnel: w345 -> [_ w355]
          frame False {
          }
          frame True {
            n218 = local write "Data Error"(w355) -> ()
            n219 = property class="Str"(reference=w357, "Value"=w356) -> ()  [unwired: 1 in, 2 out]
            n220 = local write "Msg"(w356) -> ()
          }
        }
      }
      frame #7 {
        # "Log error if COM port timeout or data error occurs."
        n221 = local read "Timeout"() -> (w393:bool)
        n222 = local read "Data Error"() -> (w389:bool)
        n223 = Index Array(array=w392, index=w394) -> (element=w402:string)
        n224 = Select(t=" Data Corrupted" ("Msg"), s=w389, f=" Data Received" ("Msg")) -> (s? t:f=w404:string)
        n225 = Select(t=" No Response at COM port" ("Msg"), s=w393, f=w404) -> (s? t:f=w400:string)
        n226 = Concatenate Strings("Unit " ("Msg"), w402) -> (w401:string)
        n227 = property class="Bool (strict)"(reference="Data Error", "Value"=w389) -> ()  [unwired: 1 in, 2 out]
        n228 = Concatenate Strings(w401, w400) -> (w391:string)
        n229 = Concatenate Strings(w391, "\r\n") -> (w396:string)
        n230 = Or(x=w393, y=w389) -> (x .or. y?=w395:bool)
        n231 = case shown="True" w395 {
          tunnel: w396 -> [_ w415]
          tunnel: w394 -> [w407 w414]
          tunnel: [w406 w410] -> w387
          frame False {
            n232 = local read "Module Error"() -> (w409:bool[])
            n233 = Replace Array Subset(array=w409, new element=FALSE ("new element/subarray"), index=w407) -> (w406:bool[])
          }
          frame True {
            w416 = "\t"
            w421 = "" ("replace string (\"\")")
            w422 = "\r\n"
            n234 = local read "Module Error"() -> (w426:bool[])
            n235 = Get Date/Time In Seconds() -> (seconds since 1Jan1904=w430:timestamp)
            n236 = Format Date/Time String(time format string (%c)="%m/%d/%y", seconds (now)=w430) -> (date/time string=w424:string)  [unwired: 1 in]
            n237 = Format Date/Time String(time format string (%c)="%H:%M:%S", seconds (now)=w430) -> (date/time string=w423:string)  [unwired: 1 in]
            n238 = Replace Array Subset(array=w426, new element=TRUE ("new element/subarray"), index=w414) -> (w410:bool[])
            n239 = local read "Error Log Msg"() -> (w433:string)
            n240 = Search and Replace String(input string=w424, search string=w422, replace string=w421) -> (result string=w418:string)  [unwired: 5 in, 3 out]
            n241 = Search and Replace String(input string=w423, search string=w422, replace string=w421) -> (result string=w417:string)  [unwired: 5 in, 3 out]
            n242 = Build Array(w418, w416, w417, w416, w415) -> (w419:string[])
            n243 = Concatenate Strings(w433, w419) -> (w411:string)
            "Error Log Msg" <- w411
            n244 = Wait Until Next ms Multiple(millisecond multiple=u32 300) -> ()  [unwired: 1 out]
            n245 = property class="Str"(reference="Error Log Msg", "Value"=w411) -> ()  [unwired: 1 in, 2 out]
            n246 = call-poly <vilib>:"Write Delimited Spreadsheet.vi"("file path (dialog if empty)"="Log File", "1D data"=w419, "append to file? (new file:F)"=TRUE ("transpose? (no:F)"), "transpose? (no:F)"=TRUE ("append to file? (new file:F)"), "delimiter (\\t)"="," ("delimiter (\\t)")) -> ()  [unwired: 9 in, 2 out]
          }
        }
        "Module Error" <- w387
        n247 = property class="Arr (strict)"(reference="Module Error", "Value"=w387) -> ()  [unwired: 1 in, 2 out]
      }
      frame #8 {
        n248 = local read "Msg"() -> (w438:string)
        n249 = Match Pattern(string=w438, regular expression="Failed") -> (offset past match=w437:i32)  [unwired: 1 in, 3 out]
        n250 = Greater Than 0?(x=w437) -> (x > 0?=w436:bool)
        n251 = Select(t=w438, s=w436, f="Reading Power Meter" ("Msg")) -> (s? t:f=w440:string)
        n252 = property class="Str"(reference=w434, "Value"=w440) -> ()  [unwired: 1 in, 2 out]
        n253 = local write "Msg"(w440) -> ()
      }
      frame #9 {
        # "Channel Select"
        # "Ch2"
        # "Ch1"
        # "Read PM"
        n254 = Quotient & Remainder(x=w442, y=2) -> (x-y*floor(x/y)=w449:i32, floor(x/y)=w443:i32)
        n255 = local read "error"() -> (w462:errorcluster)
        n256 = Increment(x=w443) -> (x+1=w444:i32)
        n257 = call "NewPort_PM_USB_Read-Set.vi"("reference"=w441, "USB Address"=w444, "Read Power(F)\nSet Lambda(T)"=FALSE ("Read Power(T)\nSet Lambda(F)"), "error in"=w462, "Read Power\nSingle CH(F)\nDual CHs(T)"=TRUE ("Set Lambda\nSingle CH(F)\nDual CHs(T)")) -> ("Query-String Format\nfrom Read Buffer"=w459:string, "error out"=w453:errorcluster)  [unwired: 9 in]
        n258 = local write "error"(w453) -> ()
        n259 = Number To Boolean Array(number=w449) -> (Boolean array=w448:bool[])
        n260 = Index Array(array=w448, index=0) -> (element=w446:bool)
        n261 = Match Pattern(string=w459, regular expression=",") -> (before substring=w458:string, after substring=w457:string)  [unwired: 1 in, 2 out]
        n262 = Not(x=w446) -> (.not. x?=w445:bool)
        n263 = Fract/Exp String To Number(string=w458) -> (number=w452:dbl)  [unwired: 3 in, 1 out]
        n264 = Fract/Exp String To Number(string=w457) -> (number=w451:dbl)  [unwired: 3 in, 1 out]
        n265 = Select(t=w452, s=w445, f=w451) -> (s? t:f=w454:dbl)
        n266 = local read "System Data"() -> (w463:dbl[])
        n267 = Build Array (concatenate)(w463, w454) -> (w455:dbl[])
        n268 = local write "System Data"(w455) -> ()
      }
      frame #10 {
        n269 = local read "Msg"() -> (w469:string)
        n270 = Match Pattern(string=w469, regular expression="Failed") -> (offset past match=w468:i32)  [unwired: 1 in, 3 out]
        n271 = Greater Than 0?(x=w468) -> (x > 0?=w467:bool)
        n272 = Select(t=w469, s=w467, f="Reading Temperature" ("Msg")) -> (s? t:f=w470:string)
        n273 = property class="Str"(reference=w465, "Value"=w470) -> ()  [unwired: 1 in, 2 out]
        n274 = local write "Msg"(w470) -> ()
      }
      frame #11 {
        # "Get Temp"
        n275 = Concatenate Strings(w471, "Mod4" ("string")) -> (w472:string)
        n276 = call "DAQ Assistant"("device name"=w472) -> ("data"=w474:dynamicdata)  [unwired: 16 in, 2 out]
        n277 = Split Signals(w474) -> (w481:dynamicdata, w479:dynamicdata, w478:dynamicdata, w473:dynamicdata)  [unwired: 4 in]
        n278 = call "Convert from Dynamic Data"("Dynamic Data Type"=w481) -> ("Array"=w480:dbl[])  [unwired: 3 in]
        n279 = call "Convert from Dynamic Data2"("Dynamic Data Type"=w479) -> ("Array"=w477:dbl[])  [unwired: 3 in]
        n280 = call "Convert from Dynamic Data3"("Dynamic Data Type"=w478) -> ("Array"=w476:dbl[])  [unwired: 3 in]
        n281 = call "Convert from Dynamic Data4"("Dynamic Data Type"=w473) -> ("Array"=w475:dbl[])  [unwired: 3 in]
        n282 = call-poly <vilib>:"Mean.vi"("X"=w480) -> ("mean"=w486:dbl)  [unwired: 1 out]
        n283 = call-poly <vilib>:"Mean.vi"("X"=w477) -> ("mean"=w485:dbl)  [unwired: 1 out]
        n284 = call-poly <vilib>:"Mean.vi"("X"=w476) -> ("mean"=w484:dbl)  [unwired: 1 out]
        n285 = call-poly <vilib>:"Mean.vi"("X"=w475) -> ("mean"=w483:dbl)  [unwired: 1 out]
        n286 = local read "System Data"() -> (w488:dbl[])
        n287 = Build Array (concatenate)(w488, w486, w485, w484, w483) -> (w487:dbl[])
        n288 = local write "System Data"(w487) -> ()
      }
      frame #12 {
        n289 = local read "Msg"() -> (w494:string)
        n290 = Match Pattern(string=w494, regular expression="Failed") -> (offset past match=w493:i32)  [unwired: 1 in, 3 out]
        n291 = Greater Than 0?(x=w493) -> (x > 0?=w492:bool)
        n292 = Select(t=w494, s=w492, f="Reading DAQ data" ("Msg")) -> (s? t:f=w495:string)
        n293 = property class="Str"(reference=w489, "Value"=w495) -> ()  [unwired: 1 in, 2 out]
        n294 = local write "Msg"(w495) -> ()
      }
      frame #13 {
        # "Get DAQ data"
        n295 = case shown="0, Default" w496 {
          tunnel: [w538 w542 w543 w547 w554 w558 w559 w563] -> w514
          frame 0, Default {
            n296 = local read "cDAQ1"() -> (w537:string)
            n297 = Concatenate Strings(w537, "Mod3" ("string")) -> (w535:string)
            n298 = call "DAQ Assistant2"("device name"=w535) -> ("data"=w538:dynamicdata)  [unwired: 16 in, 2 out]
          }
          frame 1 {
            n299 = local read "cDAQ1"() -> (w541:string)
            n300 = Concatenate Strings(w541, "Mod3" ("string")) -> (w539:string)
            n301 = call "DAQ Assistant3"("device name"=w539) -> ("data"=w542:dynamicdata)  [unwired: 16 in, 2 out]
          }
          frame 2 {
            n302 = local read "cDAQ1"() -> (w546:string)
            n303 = Concatenate Strings(w546, "Mod2" ("string")) -> (w544:string)
            n304 = call "DAQ Assistant4"("device name"=w544) -> ("data"=w543:dynamicdata)  [unwired: 16 in, 2 out]
          }
          frame 3 {
            n305 = local read "cDAQ1"() -> (w550:string)
            n306 = Concatenate Strings(w550, "Mod2" ("string")) -> (w548:string)
            n307 = call "DAQ Assistant5"("device name"=w548) -> ("data"=w547:dynamicdata)  [unwired: 16 in, 2 out]
          }
          frame 4 {
            n308 = local read "cDAQ2"() -> (w553:string)
            n309 = Concatenate Strings(w553, "Mod3" ("string")) -> (w551:string)
            n310 = call "DAQ Assistant6"("device name"=w551) -> ("data"=w554:dynamicdata)  [unwired: 16 in, 2 out]
          }
          frame 5 {
            n311 = local read "cDAQ2"() -> (w557:string)
            n312 = Concatenate Strings(w557, "Mod3" ("string")) -> (w555:string)
            n313 = call "DAQ Assistant7"("device name"=w555) -> ("data"=w558:dynamicdata)  [unwired: 16 in, 2 out]
          }
          frame 6 {
            n314 = local read "cDAQ2"() -> (w562:string)
            n315 = Concatenate Strings(w562, "Mod2" ("string")) -> (w560:string)
            n316 = call "DAQ Assistant8"("device name"=w560) -> ("data"=w559:dynamicdata)  [unwired: 16 in, 2 out]
          }
          frame 7 {
            n317 = local read "cDAQ2"() -> (w566:string)
            n318 = Concatenate Strings(w566, "Mod2" ("string")) -> (w564:string)
            n319 = call "DAQ Assistant9"("device name"=w564) -> ("data"=w563:dynamicdata)  [unwired: 16 in, 2 out]
          }
        }
        n320 = Split Signals(w514) -> (w516:dynamicdata, w518:dynamicdata, w519:dynamicdata, w520:dynamicdata, w509:dynamicdata, w506:dynamicdata, w507:dynamicdata, w508:dynamicdata)  [unwired: 8 in]
        n321 = call "Convert from Dynamic Data5"("Dynamic Data Type"=w516) -> ("Array"=w517:dbl[])  [unwired: 3 in]
        n322 = call "Convert from Dynamic Data6"("Dynamic Data Type"=w518) -> ("Array"=w521:dbl[])  [unwired: 3 in]
        n323 = call "Convert from Dynamic Data7"("Dynamic Data Type"=w519) -> ("Array"=w522:dbl[])  [unwired: 3 in]
        n324 = call "Convert from Dynamic Data8"("Dynamic Data Type"=w520) -> ("Array"=w523:dbl[])  [unwired: 3 in]
        n325 = call "Convert from Dynamic Data9"("Dynamic Data Type"=w509) -> ("Array"=w513:dbl[])  [unwired: 3 in]
        n326 = call "Convert from Dynamic Data10"("Dynamic Data Type"=w506) -> ("Array"=w512:dbl[])  [unwired: 3 in]
        n327 = call "Convert from Dynamic Data11"("Dynamic Data Type"=w507) -> ("Array"=w511:dbl[])  [unwired: 3 in]
        n328 = call "Convert from Dynamic Data12"("Dynamic Data Type"=w508) -> ("Array"=w510:dbl[])  [unwired: 3 in]
        n329 = call-poly <vilib>:"Mean.vi"("X"=w517) -> ("mean"=w532:dbl)  [unwired: 1 out]
        n330 = call-poly <vilib>:"Mean.vi"("X"=w521) -> ("mean"=w497:dbl)  [unwired: 1 out]
        n331 = call-poly <vilib>:"Mean.vi"("X"=w522) -> ("mean"=w530:dbl)  [unwired: 1 out]
        n332 = call-poly <vilib>:"Mean.vi"("X"=w523) -> ("mean"=w498:dbl)  [unwired: 1 out]
        n333 = call-poly <vilib>:"Mean.vi"("X"=w513) -> ("mean"=w528:dbl)  [unwired: 1 out]
        n334 = call-poly <vilib>:"Mean.vi"("X"=w512) -> ("mean"=w499:dbl)  [unwired: 1 out]
        n335 = call-poly <vilib>:"Mean.vi"("X"=w511) -> ("mean"=w500:dbl)  [unwired: 1 out]
        n336 = call-poly <vilib>:"Mean.vi"("X"=w510) -> ("mean"=w501:dbl)  [unwired: 1 out]
        n337 = Multiply(x=w497, y=0.25 ("mean")) -> (x*y=w531:dbl)
        n338 = Multiply(x=w498, y=0.25 ("mean")) -> (x*y=w529:dbl)
        n339 = Multiply(x=w499, y=0.25 ("mean")) -> (x*y=w527:dbl)
        n340 = Multiply(x=w500, y=5.814 ("mean")) -> (x*y=w526:dbl)
        n341 = Multiply(x=w501, y=0.25 ("mean")) -> (x*y=w525:dbl)
        n342 = Build Array(w532, w531, w530, w529, w528, w527, w526, w525) -> (w524:dbl[])
        n343 = local read "System Data"() -> (w534:dbl[])
        n344 = Build Array (concatenate)(w534, w524) -> (w533:dbl[])
        n345 = local write "System Data"(w533) -> ()
      }
      frame #14 {
        # "Take optical power readings if shutter open time met minimum duration requirement."
        n346 = case shown="True" w571 {
          tunnel: w573 -> [_ w582]
          tunnel: w572 -> [_ w581]
          tunnel: w570 -> [_ w580]
          tunnel: w569 -> [_ w579]
          tunnel: w568 -> [_ w578]
          tunnel: w567 -> [_ w577]
          frame False {
            # "If required time duration for open shutter not met, use zero value as place holder for closed shutter power reading."
            n347 = local read "System Data"() -> (w574:dbl[])
            n348 = Build Array (concatenate)(w574, 0.0 ("element")) -> (w576:dbl[])
            n349 = local write "System Data"(w576) -> ()
          }
          frame True {
            n350 = stacked-sequence {
              tunnel: w582 -> [w590 _ _ w620 _ w667]
              tunnel: w581 -> [_ _ _ w619 _ _]
              tunnel: w580 -> [_ _ w615 _ _ _]
              tunnel: w579 -> [_ _ _ _ w644 _]
              tunnel: w578 -> [_ _ _ _ w643 _]
              tunnel: w577 -> [w583 _ _ _ _ w659]
              frame #0 {
                w591 = 4 ("y")
                w594 = FALSE
                # "F=open, T=closed"
                # "Close shutter individually with respect to the particular unit under test."
                n351 = Build Array(w594, w594, w594, w594) -> (w593:bool[])
                n352 = Greater Or Equal?(x=w590, y=w591) -> (x >= y?=w592:bool)
                n353 = case shown="False" w592 {
                  tunnel: w590 -> [w597 w604]
                  tunnel: w593 -> [w599 w606]
                  tunnel: w591 -> [w596 _]
                  frame True {
                    n354 = Subtract(x=w597, y=w596) -> (x-y=w595:i32)
                    n355 = Replace Array Subset(array=w599, new element=TRUE, index=w595) -> (w598:bool[])
                    n356 = local read "cDAQ2"() -> (w601:string)
                    n357 = Concatenate Strings(w601, "Mod1" ("string")) -> (w603:string)
                    n358 = call "DAQ Assistant10"("data"=w598, "device name"=w603) -> ()  [unwired: 16 in, 2 out]
                  }
                  frame False {
                    n359 = Replace Array Subset(array=w606, new element=TRUE, index=w604) -> (w605:bool[])
                    n360 = local read "cDAQ1"() -> (w608:string)
                    n361 = Concatenate Strings(w608, "Mod1" ("string")) -> (w610:string)
                    n362 = call "DAQ Assistant11"("data"=w605, "device name"=w610) -> ()  [unwired: 16 in, 2 out]
                  }
                }
                n363 = local read "Msg"() -> (w588:string)
                n364 = Match Pattern(string=w588, regular expression="Failed") -> (offset past match=w587:i32)  [unwired: 1 in, 3 out]
                n365 = Greater Than 0?(x=w587) -> (x > 0?=w586:bool)
                n366 = Select(t=w588, s=w586, f="Cycle shutter to take PM data." ("Msg")) -> (s? t:f=w589:string)
                n367 = property class="Str"(reference=w583, "Value"=w589) -> ()  [unwired: 1 in, 2 out]
                n368 = local write "Msg"(w589) -> ()
              }
              frame #1 {
                w612 = FALSE ("Sttrs Open")
                w611 = TRUE ("Sttrs Close")
                # "Update calling VI indicators"
                # "No need to pass this indicator value to calling VI."
                # "No need to pass this indicator value to calling VI."
                n369 = property class="Bool (strict)"(reference="Shutter Opened", "Value"=w611) -> ()  [unwired: 1 in, 2 out]
                n370 = local write "Shtr Close"(w611) -> ()
                n371 = property class="Bool (strict)"(reference="Shutter Closed", "Value"=w612) -> ()  [unwired: 1 in, 2 out]
                n372 = local write "Shtr Open"(w612) -> ()
              }
              frame #2 {
                # "Close shutter for specified interval."
                n373 = To Unsigned Long Integer(number=w615) -> (unsigned 32bit integer=w616:u32)
                n374 = Multiply(x=w616, y=u32 1000 ("milliseconds to wait")) -> (x*y=w618:u32)
                n375 = Wait (ms)(milliseconds to wait=w618) -> ()  [unwired: 1 out]
              }
              frame #3 {
                # "Channel Select"
                # "Ch2"
                # "Ch1"
                # "USB-read power meter while shutter closed."
                n376 = Quotient & Remainder(x=w620, y=2) -> (x-y*floor(x/y)=w631:i32, floor(x/y)=w622:i32)
                n377 = local read "error"() -> (w640:errorcluster)
                n378 = Increment(x=w622) -> (x+1=w621:i32)
                n379 = call "NewPort_PM_USB_Read-Set.vi"("reference"=w619, "USB Address"=w621, "Read Power(F)\nSet Lambda(T)"=FALSE ("Read Power(T)\nSet Lambda(F)"), "error in"=w640, "Read Power\nSingle CH(F)\nDual CHs(T)"=TRUE ("Set Lambda\nSingle CH(F)\nDual CHs(T)")) -> ("Query-String Format\nfrom Read Buffer"=w639:string, "error out"=w634:errorcluster)  [unwired: 9 in]
                n380 = Number To Boolean Array(number=w631) -> (Boolean array=w630:bool[])
                n381 = local write "error"(w634) -> ()
                n382 = Index Array(array=w630, index=0) -> (element=w629:bool)
                n383 = Match Pattern(string=w639, regular expression=",") -> (before substring=w638:string, after substring=w637:string)  [unwired: 1 in, 2 out]
                n384 = Not(x=w629) -> (.not. x?=w628:bool)
                n385 = Fract/Exp String To Number(string=w638) -> (number=w633:dbl)  [unwired: 3 in, 1 out]
                n386 = Fract/Exp String To Number(string=w637) -> (number=w632:dbl)  [unwired: 3 in, 1 out]
                n387 = Select(t=w633, s=w628, f=w632) -> (s? t:f=w635:dbl)
                n388 = local read "System Data"() -> (w641:dbl[])
                n389 = Build Array (concatenate)(w641, w635) -> (w636:dbl[])
                n390 = local write "System Data"(w636) -> ()
              }
              frame #4 {
                w650 = FALSE
                # "No need to pass this indicator value to calling VI."
                # "No need to pass this indicator value to calling VI."
                # "F=open, T=closed"
                n391 = Build Array(w650, w650, w650, w650) -> (w649:bool[])
                n392 = local read "UUT Count"() -> (w648:i32)
                n393 = Greater?(x=w648, y=4) -> (0:w646:bool)
                n394 = case shown="True" w646 {
                  tunnel: w649 -> [w652 w656]
                  tunnel: w644 -> [_ w655]
                  tunnel: w643 -> [w651 _]
                  frame True {
                    n395 = Concatenate Strings(w651, "Mod1" ("string")) -> (w654:string)
                    n396 = call "DAQ Assistant12"("data"=w652, "device name"=w654) -> ()  [unwired: 16 in, 2 out]
                  }
                  frame False {
                    n397 = Concatenate Strings(w655, "Mod1" ("string")) -> (w658:string)
                    n398 = call "DAQ Assistant13"("data"=w656, "device name"=w658) -> ()  [unwired: 16 in, 2 out]
                  }
                }
                "Shtr Open" <- TRUE ("Sttrs Open")
                "Shtr Close" <- FALSE ("Sttrs Close")
              }
              frame #5 {
                # "Update the start time of shutter open after data collected for all units in this particular sample."
                n399 = local read "UUT Count"() -> (w669:i32)
                n400 = Increment(x=w667) -> (x+1=w666:i32)
                n401 = local read "Msg"() -> (w664:string)
                n402 = Greater Or Equal?(x=w666, y=w669) -> (x >= y?=w668:bool)
                n403 = case shown="True" w668 {
                  frame False {
                  }
                  frame True {
                    # "Not necessary to toggle this Boolean if\nperformed in calling VI after execution."
                    n404 = local read "Data Time"() -> (w670:timestamp)
                    n405 = local write "Tpass Shtr Open"(FALSE ("Pass 3 Minute")) -> ()
                    n406 = local write "Shtr Ref Time"(w670) -> ()
                  }
                }
                n407 = Match Pattern(string=w664, regular expression="Failed") -> (offset past match=w663:i32)  [unwired: 1 in, 3 out]
                n408 = Greater Than 0?(x=w663) -> (x > 0?=w662:bool)
                n409 = Select(t=w664, s=w662, f="Save and process collected data." ("Msg")) -> (s? t:f=w665:string)
                n410 = property class="Str"(reference=w659, "Value"=w665) -> ()  [unwired: 1 in, 2 out]
                n411 = local write "Msg"(w665) -> ()
              }
            }
          }
        }
      }
      frame #15 {
        # "\"Meas N\" equals sum total of UUT and system paparameter count +1 (for time)."
        # "Keeps track of # of\ndata samples for\neach UUT."
        n412 = local read "All Results"() -> (w677:dbl[][][])
        n413 = local read "Points"() -> (w679:i32[])
        n414 = Array Size(array=w677) -> (size(s)=w674:i32[])
        n415 = Index Array(array=w679, index=w673) -> (element=w682:i32)
        n416 = Increment(x=w682) -> (x+1=w680:i32)
        n417 = Replace Array Subset(array=w679, new element=w680, index=w673) -> (w681:i32[])
        n418 = local write "Points"(w681) -> ()
        n419 = Index Array(array=w674, index=1) -> (element=w676:i32)
        n420 = Greater?(x=w680, y=w676) -> (0:w678:bool)
        n421 = case shown="True" w678 {
          tunnel: w677 -> [_ w689]
          tunnel: w682 -> [_ w688]
          tunnel: w672 -> [_ w683]
          frame False {
          }
          frame True {
            # "Equivalent to using \"Build Array\" to expand the \"All Results\" array incrementally as needed when  number of acquired data points exceeds previous allocation."
            n422 = local read "UUT Count"() -> (w687:i32)
            n423 = Initialize Array(0.0 ("element"), w687, w683) -> (w685:dbl[][])
            n424 = Insert Into Array(array=w689, index (dim 1)=w688, new element=w685) -> (w684:dbl[][][])  [unwired: 2 in]
            n425 = local write "All Results"(w684) -> ()
          }
        }
      }
      frame #16 {
        # "Store newly acquired MCU and System Data to All Results Array."
        # "\"All Results\" Local Variable Indice Definition:\n0 = Unit #\n1 = Sample #\n2 = Parameter Values"
        n426 = local read "All Results"() -> (w697:dbl[][][])
        n427 = local read "Points"() -> (w698:i32[])
        n428 = local read "Data Time"() -> (w695:timestamp)
        n429 = local read "MCU Data"() -> (w691:dbl[])
        n430 = local read "System Data"() -> (w690:dbl[])
        n431 = To Double Precision Float(number=w695) -> (double precision float=w694:dbl)
        n432 = Index Array(array=w698, index=w693) -> (element=w699:i32)
        n433 = Build Array (concatenate)(w694, w691, w690) -> (w696:dbl[])
        n434 = Decrement(x=w699) -> (x-1=w700:i32)
        n435 = Replace Array Subset(array=w697, new element=w696, index (dim 0)=w693, index (dim 1)=w700) -> (→"All Results":dbl[][][])  [unwired: 1 in]
      }
      frame #17 {
        # "Pass: Green (F); \nFail:  Yellow (T)"
        # "max"
        # "min"
        # "Pass: Green (F); \nFail:  Yellow (T)"
        # "max"
        # "min"
        # "Criteria check of test data."
        n436 = Index Array(array=w701, index (col)=1 ("disabled index (col)")) -> (element=w712:string[])  [unwired: 1 in]
        n437 = Index Array(array=w701, index (col)=0 ("disabled index (col)")) -> (element=w713:string[])  [unwired: 1 in]
        n438 = Index Array(array=w702, index (col)=1 ("disabled index (col)")) -> (element=w705:string[])  [unwired: 1 in]
        n439 = Index Array(array=w702, index (col)=0 ("disabled index (col)")) -> (element=w704:string[])  [unwired: 1 in]
        n440 = Array Size(array=w705) -> (size(s)=w706:i32)
        n441 = Array Size(array=w712) -> (size(s)=w711:i32)
        n442 = for {
          N: w711 -> [_]
          tunnel: w712 -> [w740] mode=indexing
          tunnel: w713 -> [w738] mode=indexing
          tunnel: w703 -> [w731]
          i -> [w732]
          # "delete time"
          n443 = local read "MCU Data"() -> (w743:dbl[])
          n444 = local read "MCUTrue"() -> (w730:bool[][])
          n445 = Scan Value(string=w740, format string="%9.6f") -> (value=w739:dbl)  [unwired: 1 in, 1 out]
          n446 = Index Array(array=w743, index=w732) -> (element=w742:dbl)
          n447 = Scan Value(string=w738, format string="%9.6f") -> (value=w736:dbl)  [unwired: 1 in, 1 out]
          n448 = Index Array(array=w730, index (row)=w732, index (col)=w731) -> (element=w735:bool)
          n449 = In Range and Coerce(upper limit=w739, x=w742, lower limit=w736) -> (In Range?=w733:bool)  [unwired: 1 out]
          n450 = And(x=w733, y=w735) -> (x .and. y?=w734:bool)
          n451 = Replace Array Subset(array=w730, new element=w734, index (row)=w732, index (col)=w731) -> (→"MCUTrue":bool[][])
        }
        n452 = for {
          N: w706 -> [_]
          tunnel: w705 -> [w726] mode=indexing
          tunnel: w704 -> [w724] mode=indexing
          tunnel: w703 -> [w716]
          i -> [w717]
          n453 = local read "SysTrue"() -> (w715:bool[][])
          n454 = local read "System Data"() -> (w719:dbl[])
          n455 = Scan Value(string=w726, format string="%9.6f") -> (value=w725:dbl)  [unwired: 1 in, 1 out]
          n456 = Index Array(array=w719, index=w717) -> (element=w728:dbl)
          n457 = Scan Value(string=w724, format string="%9.6f") -> (value=w722:dbl)  [unwired: 1 in, 1 out]
          n458 = Index Array(array=w715, index (row)=w717, index (col)=w716) -> (element=w721:bool)
          n459 = In Range and Coerce(upper limit=w725, x=w728, lower limit=w722) -> (In Range?=w718:bool)  [unwired: 1 out]
          n460 = And(x=w718, y=w721) -> (x .and. y?=w720:bool)
          n461 = Replace Array Subset(array=w715, new element=w720, index (row)=w717, index (col)=w716) -> (→"SysTrue":bool[][])
        }
      }
      frame #18 {
        # "Question for Jie:  Why  use either \"R\" or no string characters for results of MCUCheck and SysCheck?  Why are these indicators needed in addition to the Boolean arrays?"
        # "7-7-17 Added, convert parameter review status from boolean to string"
        n462 = local read "MCUTrue"() -> (w745:bool[][])
        n463 = local read "SysTrue"() -> (w748:bool[][])
        n464 = Index Array(array=w748, index (col)=w744) -> (element=w747:bool[])  [unwired: 1 in]
        n465 = Index Array(array=w745, index (col)=w744) -> (element=w746:bool[])  [unwired: 1 in]
        n466 = for {
          tunnel: w746 -> [w758] mode=indexing
          tunnel: w744 -> [w761]
          i -> [w760]
          n467 = local read "MCUCheck"() -> (w762:string[][])
          n468 = Select(t="", s=w758, f="R") -> (s? t:f=w759:string)
          n469 = Replace Array Subset(array=w762, new element=w759, index (row)=w760, index (col)=w761) -> (→"MCUCheck":string[][])
        }
        n470 = for {
          tunnel: w747 -> [w756] mode=indexing
          tunnel: w744 -> [w752]
          i -> [w751]
          n471 = local read "SysCheck"() -> (w753:string[][])
          n472 = Select(t="", s=w756, f="R") -> (s? t:f=w750:string)
          n473 = Replace Array Subset(array=w753, new element=w750, index (row)=w751, index (col)=w752) -> (→"SysCheck":string[][])
        }
      }
      frame #19 {
        n474 = local write "Msg"("Idle" ("Msg")) -> ()
      }
    }
  }
  "MCU Data Array" <- w3
  "System Data Array" <- w2
  "Update Graph" <- w20
  "Save" <- w20
  "Collect" <- FALSE ("Collect")
